vi "_069.vi"() -> ()   [LabVIEW 2024]
panel:
  in  "stop":bool
  out "Waveform Chart":dbl(graph)
  # "Code will wait for users permission :"
  # "( user control without event programming )"
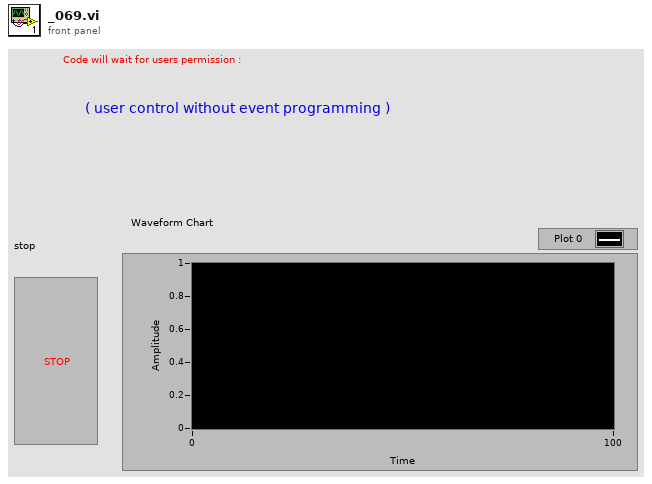
[diagram p1: front panel]
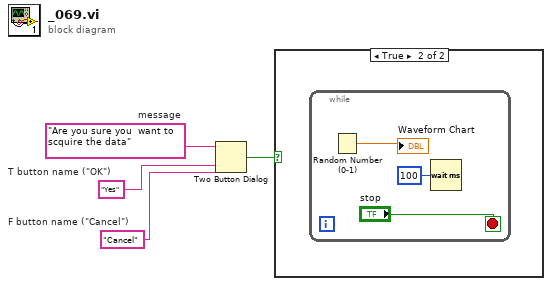
[diagram p0: block diagram]
diagram:
  w2 = "Cancel"  # F button name ("Cancel")
  w3 = "Yes"  # T button name ("OK")
  w4 = "Are you sure you  want to scquire the data"  # message
  n1 = Two Button Dialog(message=w4, 1:w2, 2:w3) -> (T button?=w1:bool)
  n2 = case shown="True" w1 {
    frame False {
    }
    frame True {
      n3 = while {
        stop <- "stop" stop-if-true
        n4 = Random Number (0-1)() -> (number: 0 to 1=→"Waveform Chart":dbl)
        n5 = Wait (ms)(milliseconds to wait=u32 100) -> ()  [unwired: 1 out]
      }
    }
  }
